vi "Construct mysql configuration database queries.vi"(4 "value column(value)":string="value", 6 "name column(name)":string="name", 8 "error in (no error)":errorcluster, 10 "table":string="configuration", 11 "database(configuration)":string="mydatabase") -> (0 "error out":errorcluster, 3 "mysql-configdb-queries out":refnum<class "mysql-queries.lvclass">)   [LabVIEW 2020, in "mysql-queries.lvlib" / "mysql-queries.lvclass"]
uses:
  mysql-queries.lvclass
  mysql-queries.lvclass/mysql-queries.ctl
  externals/database-interface/IDatabase/IDatabase.lvlib
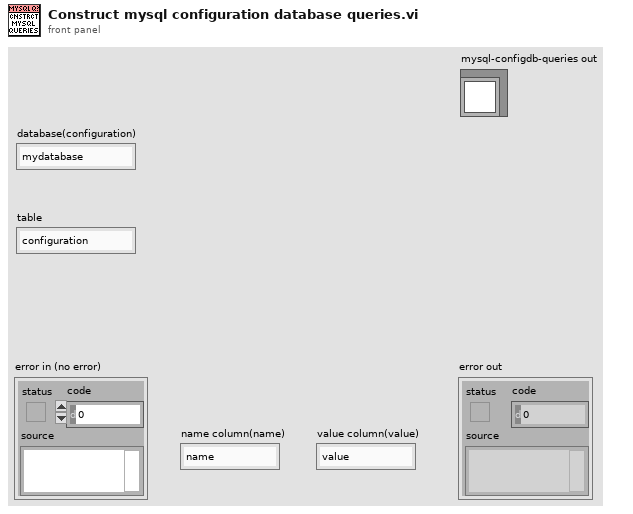
[diagram p1: front panel]
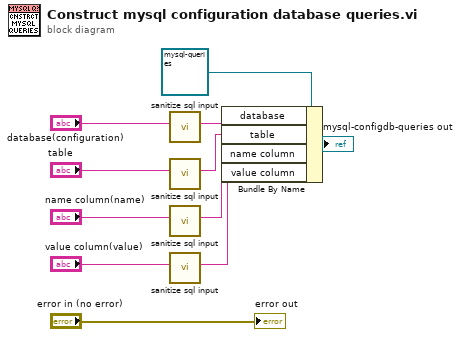
[diagram p0: block diagram]
diagram:
  n1 = call "sanitize sql input.vi"("Sting in"="database(configuration)") -> ("String out"=w4:string)  [unwired: 8 in, 2 out]
  n2 = call "sanitize sql input.vi"("Sting in"="table") -> ("String out"=w3:string)  [unwired: 8 in, 2 out]
  n3 = call "sanitize sql input.vi"("Sting in"="name column(name)") -> ("String out"=w2:string)  [unwired: 8 in, 2 out]
  n4 = call "sanitize sql input.vi"("Sting in"="value column(value)") -> ("String out"=w1:string)  [unwired: 8 in, 2 out]
  n5 = Bundle By Name(cluster=refnum<class "mysql-queries.lvclass"> refnum ("mysql-configdb-queries in"), "database"=w4, "table"=w3, "name column"=w2, "value column"=w1) -> (→"mysql-configdb-queries out":refnum<class "mysql-queries.lvclass">)
  "error out" <- "error in (no error)"
